vi "GT_GetSts.vi"(10 "Axis":T1=1 items=["Axis Control"=0, "Axis 1"=1, "Axis 2"=2, "Axis 3"=3, "Axis 4"=4, "Axis 5"=5, "Axis 6"=6, "Axis 7"=7, "Axis 8"=8, "Vector Space Control"=16, "Vector Space 1"=17, "Vector Space 2"=18, "Vector Space 3"=19, "Vector Space 4"=20], 11 "rtn_In":cluster{"rtn":i16, "Func":string}) -> (0 "DiverAlram":bool, 1 "Axis":T1 items=["Axis Control"=0, "Axis 1"=1, "Axis 2"=2, "Axis 3"=3, "Axis 4"=4, "Axis 5"=5, "Axis 6"=6, "Axis 7"=7, "Axis 8"=8, "Vector Space Control"=16, "Vector Space 1"=17, "Vector Space 2"=18, "Vector Space 3"=19, "Vector Space 4"=20], 2 "pSts":i32, 3 "rtn_Out":cluster{"rtn":i16, "Func":string}, 4 "Stop":bool, 5 "Strings":string)   [LabVIEW 2014]
uses:
  <vilib>/Motion/FlexMotion/CustomControls/CustomControls.llb/AxisOrVectorSpaceControl To Control.flx
  VC6/gts.dll
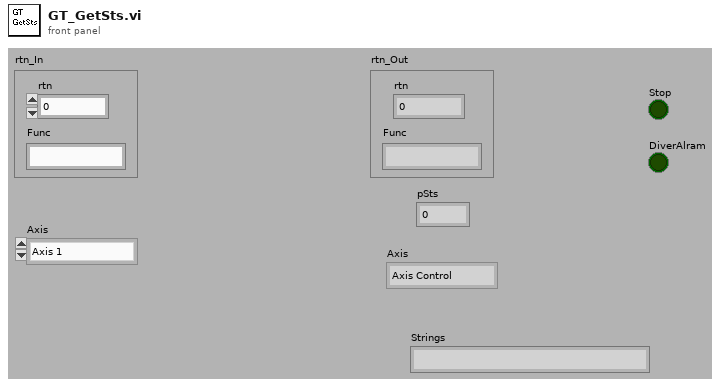
[diagram p1: front panel]
types:
  T1 = typedef "AxisOrVectorSpaceControl To Control.flx" = u16
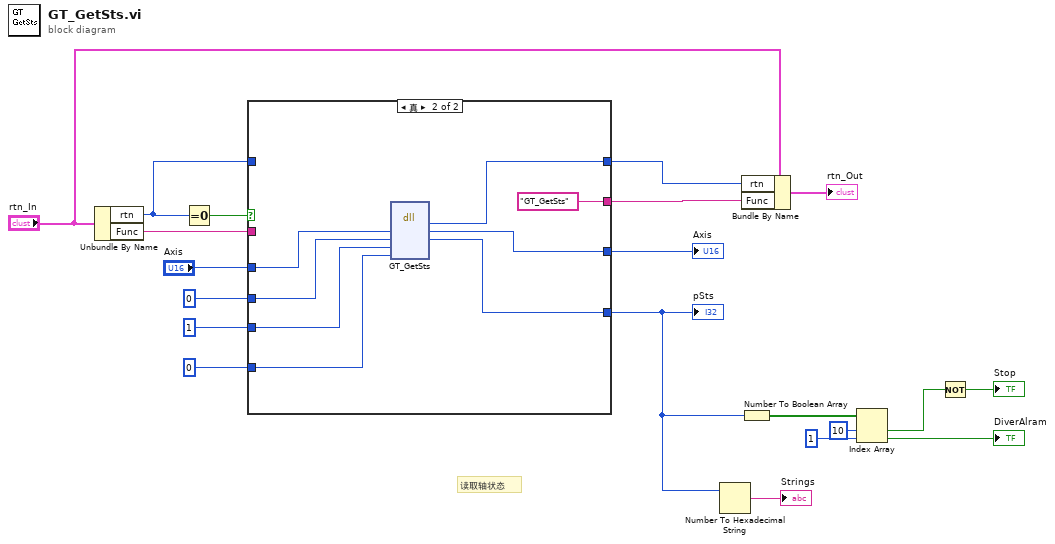
[diagram p0: block diagram]
diagram:
  # "读取轴状态"
  n1 = Unbundle By Name("rtn_In") -> ("rtn"=w15:i16, "Func"=w17:string)
  n2 = Equal To 0?(x=w15) -> (x = 0?=w20:bool)
  n3 = case shown="真" w20 {
    tunnel: [w24 "GT_GetSts" ("Func")] -> w18
    tunnel: w17 -> [w24 _]
    tunnel: [w23 w31] -> w16
    tunnel: w15 -> [w23 _]
    tunnel: "Axis" -> [w22 w30]
    tunnel: [w22 w29] -> w2
    tunnel: 0 ("pSts") -> [w21 w28]
    tunnel: i16 1 ("count") -> [_ w27]
    tunnel: u32 0 ("pClock") -> [_ w26]
    tunnel: [w21 w25] -> w5
    frame False {
    }
    frame True {
      n4 = dll-call lib="PTH2Fabs DNewGTS AC-800LWin7版源程序-20170926gts85VC6gts.dll" fn="GT_GetSts"("axis"=w30, "pSts"=w28, "count"=w27, "pClock"=w26) -> ("rtn"=w31:i16, "axis"=w29:i16, "pSts"=w25:i32)  [unwired: 5 in, 2 out]
    }
  }
  "pSts" <- w5
  "Axis" <- w2
  n5 = Number To Hexadecimal String(2:w5) -> (0:→"Strings":string)  [unwired: 1 in]
  n6 = Bundle By Name(cluster="rtn_In", "rtn"=w16, "Func"=w18) -> (→"rtn_Out":cluster{"rtn":i16, "Func":string})
  n7 = Number To Boolean Array(number=w5) -> (Boolean array=w11:bool[])
  n8 = Index Array(array=w11, index #1=10 ("索引"), index #2=1 ("索引")) -> (element #1=w8:bool, element #2=→"DiverAlram":bool)
  n9 = Not(x=w8) -> (.not. x?=→"Stop":bool)
